vi "TimerCaseVI.vi"() -> ()   [LabVIEW 2023]
panel:
  in  "Boolean 3":bool
  in  "stop":bool
  out "Numeric 2":dbl
  out "Boolean 2":bool
  in  "Numeric":dbl
  in  "Boolean":bool
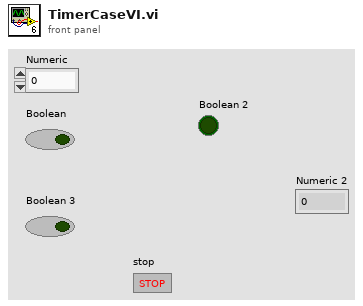
[diagram p1: front panel]
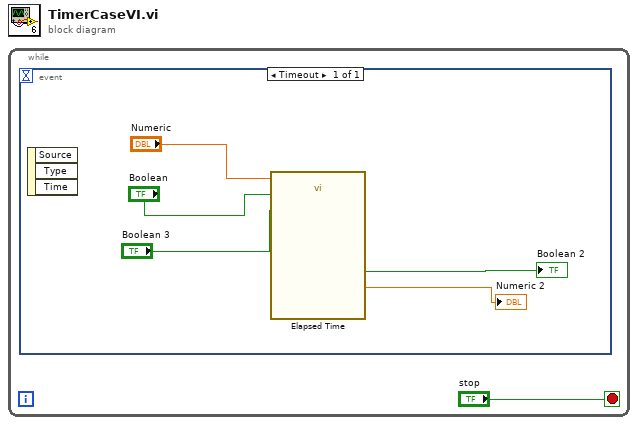
[diagram p0: block diagram]
diagram:
  n1 = while {
    stop <- "stop" stop-if-true
    n2 = event shown="[0] Timeout" {
      selector: _ -> [_]
      dyn-events: _ -> [_]
      timeout: _ -> [_]
      event Timeout {
        n3 = event-data() -> ()  [unwired: 1 in, 3 out]
        n4 = call "Elapsed Time"("Time Target (s)"="Numeric", "Reset"="Boolean", "Auto Reset"="Boolean 3") -> ("Elapsed Time (s)"=→"Numeric 2":dbl, "Time has Elapsed"=→"Boolean 2":bool)  [unwired: 9 in, 6 out]
      }
    }
  }
